vi "Admin Submissions JSON.vi"(8 "error in (no error)":errorcluster, 11 "Submission DB in":refnum<class "Submission DB.lvclass">) -> (0 "error out":errorcluster, 2 "Admin Info JSON":T1, 3 "Submission DB out":refnum<class "Submission DB.lvclass">)   [LabVIEW 2020, in "Summer of LabVIEW.lvlib" / "Submission DB.lvclass"]
uses:
  Submission DB.lvclass
  Data Types/Admin Info JSON.ctl
  Data Types/Pending Submission JSON.ctl
  Submission DB.lvclass/Submission DB.ctl
  <vilib>/drjdpowell/SQLite Library/SQL Statement/SQL Statement.lvclass/SQL Statement.ctl
  SoL Scoring/Score.ctl
  SoL Scoring/Score Entry.ctl
  <vilib>/drjdpowell/SQLite Library/SQL Statement/Column I64.vi
  <vilib>/drjdpowell/SQLite Library/SQL Statement/Error Message.vi
  <vilib>/drjdpowell/SQLite Library/SQL Statement/Column String.vi
  SQLite/SQLite.lvclass
  <vilib>/drjdpowell/SQLite Library/SQL Connection/Connection.lvclass
  <vilib>/drjdpowell/SQLite Library/SQL Statement/SQL Statement.lvclass
  Summer of LabVIEW.lvlib
  SoL Scoring/SoL Scoring.lvlib
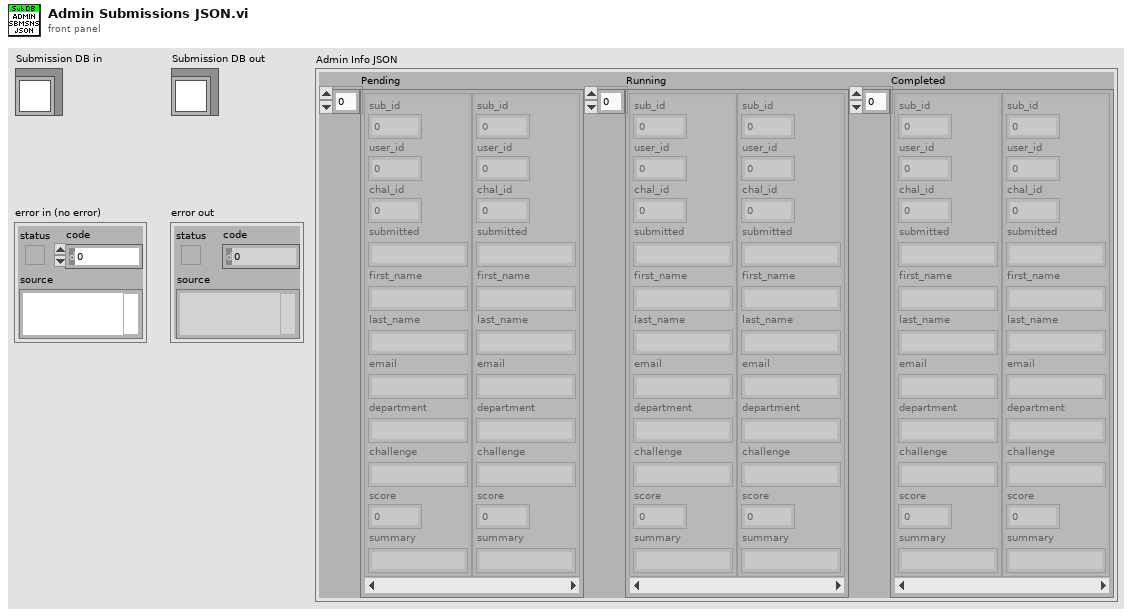
[diagram p1: front panel]
types:
  T1 = typedef "Summer of LabVIEW.lvlib/Admin Info JSON.ctl" = cluster{"Pending":T2[], "Running":T2[], "Completed":T2[]}
  T2 = typedef "Summer of LabVIEW.lvlib/Pending Submission JSON.ctl" = cluster{"sub_id":i64, "user_id":i64, "chal_id":i64, "submitted":string, "first_name":string, "last_name":string, "email":string, "department":string, "challenge":string, "score":dbl, "summary":string}
  T3 = typedef "SoL Scoring.lvlib/Score.ctl" = cluster{"Overall":dbl, "Categories":T4[]}
  T4 = typedef "SoL Scoring.lvlib/Score Entry.ctl" = cluster{"Category":string, "Value":dbl}
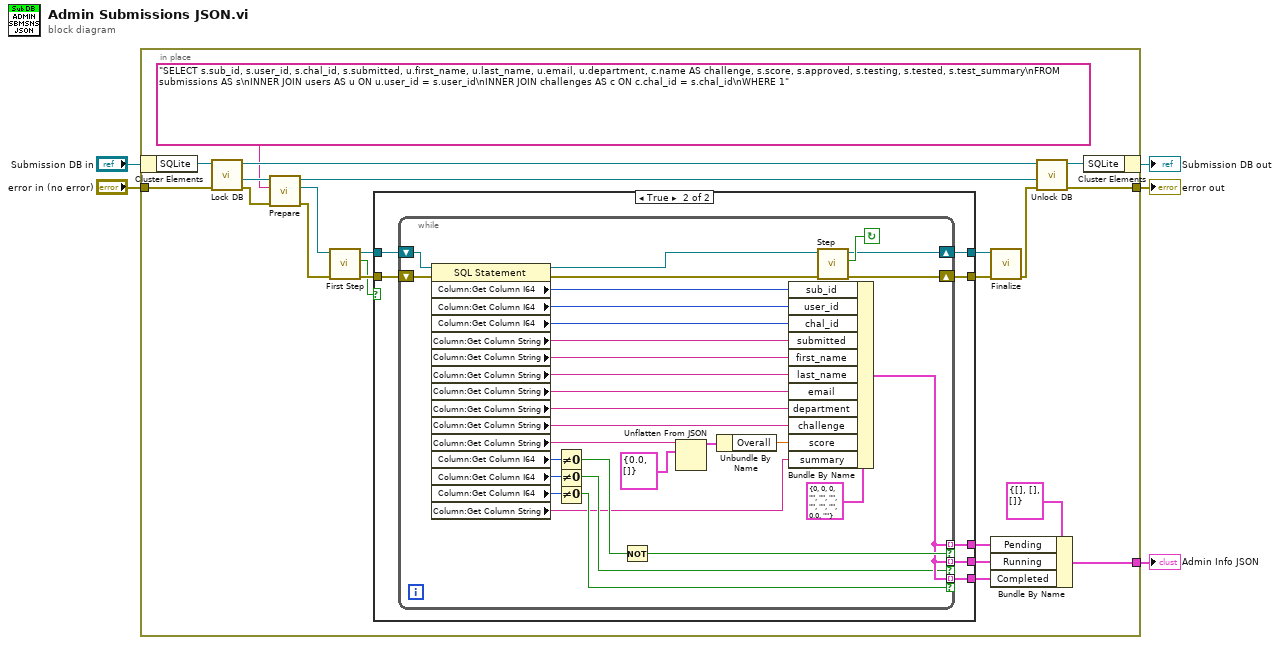
[diagram p0: block diagram]
diagram:
  n1 = in-place {
    in-place-border: "error in (no error)" -> [w26]
    in-place-border: [w23] -> w3
    in-place-border: [w6] -> w1
    n2 = in-place-cluster #1("Submission DB in") -> ("SQLite"=w27:refnum<class "SQLite.lvclass">)
    n3 = call "Lock DB.vi"("error in (no error)"=w26, "SQLite in"=w27) -> ("error out"=w19:errorcluster, "SQLite DB"=w22:refnum<class "Connection.lvclass">, "SQLite out"=w25:refnum<class "SQLite.lvclass">)  [unwired: 6 in, 1 out]
    n4 = call <vilib>:"Prepare.vi"("error in (no error)"=w19, "SQL"="SELECT s.sub_id, s.user_id, s.chal_id, s.submitted, u.first_name, u.last_name, u.email, u.department, c.name AS challenge, s.score, s.approved, s.testing, s.tested, s.test_summary\nFROM submissions AS s\nINNER JOIN users AS u ON u.user_id = s.user_id\nINNER JOIN challenges AS c ON c.chal_id = s.chal_id\nWHERE 1", "SQLite Connection in"=w22) -> ("error out"=w18:errorcluster, "SQL Statement"=w20:refnum<class "SQL Statement.lvclass">, "SQLite Connection"=w11:refnum<class "Connection.lvclass">)  [unwired: 4 in, 2 out]
    n5 = call <vilib>:"First Step.vi"("error in (no error)"=w18, "SQL Statement in"=w20) -> ("error out"=w17:errorcluster, "Row returned"=w16:bool, "SQL Statement"=w15:refnum<class "SQL Statement.lvclass">)  [unwired: 7 in]
    n6 = case shown="True" w16 {
      tunnel: w17 -> [w28 w35]
      tunnel: w15 -> [w29 w36]
      tunnel: [w29 w34] -> w14
      tunnel: [w28 w33] -> w13
      tunnel: [_ w32] -> w9
      tunnel: [_ w31] -> w8
      tunnel: [_ w30] -> w7
      frame False {
      }
      frame True {
        n7 = while {
          shift-right: [w60] -> w34
          shift-left: w36 -> [w65]
          shift-right: [w63] -> w33
          shift-left: w35 -> [w66]
          tunnel: [w40] -> w32 mode=indexing if=w41
          tunnel: [w40] -> w31 mode=indexing if=w39
          tunnel: [w40] -> w30 mode=indexing if=w38
          stop <- w62 continue-if-true
          n8 = property class="SQL Statement"(reference=w65, error in=w66) -> (reference out=w61:refnum<class "SQL Statement.lvclass">, error out=w64:errorcluster, "Column:Get Column I64"=w58:i64, "Column:Get Column I64"=w57:i64, "Column:Get Column I64"=w56:i64, "Column:Get Column String"=w55:string, "Column:Get Column String"=w54:string, "Column:Get Column String"=w53:string, "Column:Get Column String"=w52:string, "Column:Get Column String"=w51:string, "Column:Get Column String"=w50:string, "Column:Get Column String"=w49:string, "Column:Get Column I64"=w45:i64, "Column:Get Column I64"=w44:i64, "Column:Get Column I64"=w43:i64, "Column:Get Column String"=w37:string)
          n9 = Not Equal To 0?(x=w45) -> (x != 0?=w42:bool)
          n10 = Not Equal To 0?(x=w44) -> (x != 0?=w39:bool)
          n11 = Not Equal To 0?(x=w43) -> (x != 0?=w38:bool)
          n12 = Not(x=w42) -> (.not. x?=w41:bool)
          n13 = Unflatten From JSON(JSON string=w49, type and defaults=T3 {"Overall"=0.0, "Categories"=[]} ("Score")) -> (value=w47:T3)  [unwired: 5 in, 1 out]
          n14 = Unbundle By Name(w47) -> ("Overall"=w46:dbl)
          n15 = Bundle By Name(cluster=T2 {"sub_id"=0, "user_id"=0, "chal_id"=0, "submitted"="", "first_name"="", "last_name"="", "email"="", "department"="", "challenge"="", "score"=0.0, "summary"=""} ("Pending Submission JSON"), "sub_id"=w58, "user_id"=w57, "chal_id"=w56, "submitted"=w55, "first_name"=w54, "last_name"=w53, "email"=w52, "department"=w51, "challenge"=w50, "score"=w46, "summary"=w37) -> (w40:T2)
          n16 = call <vilib>:"Step.vi"("error in (no error)"=w64, "SQL Statement in"=w61) -> ("error out"=w63:errorcluster, "Row returned"=w62:bool, "SQL Statement"=w60:refnum<class "SQL Statement.lvclass">)  [unwired: 7 in]
        }
      }
    }
    n17 = call <vilib>:"Finalize.vi"("error in (no error)"=w13, "SQL Statement in"=w14) -> ("error out"=w12:errorcluster)  [unwired: 9 in]
    n18 = Bundle By Name(cluster=T1 {"Pending"=[], "Running"=[], "Completed"=[]} ("Admin Info JSON"), "Pending"=w9, "Running"=w8, "Completed"=w7) -> (w6:T1)
    n19 = call "Unlock DB.vi"("error in (no error)"=w12, "SQLite DB"=w11, "SQLite in"=w25) -> ("error out"=w23:errorcluster, "SQLite out"=w24:refnum<class "SQLite.lvclass">)  [unwired: 7 in]
    n20 = in-place-cluster #1("SQLite"=w24) -> (→"Submission DB out":refnum<class "Submission DB.lvclass">)
  }
  "error out" <- w3
  "Admin Info JSON" <- w1
